vi "senser.vi"(1 "read buffer":string) -> (0 "输出簇":cluster{"T1":i16, "T2":i16, "T3":i16, "T4":i16})   [LabVIEW 2014]
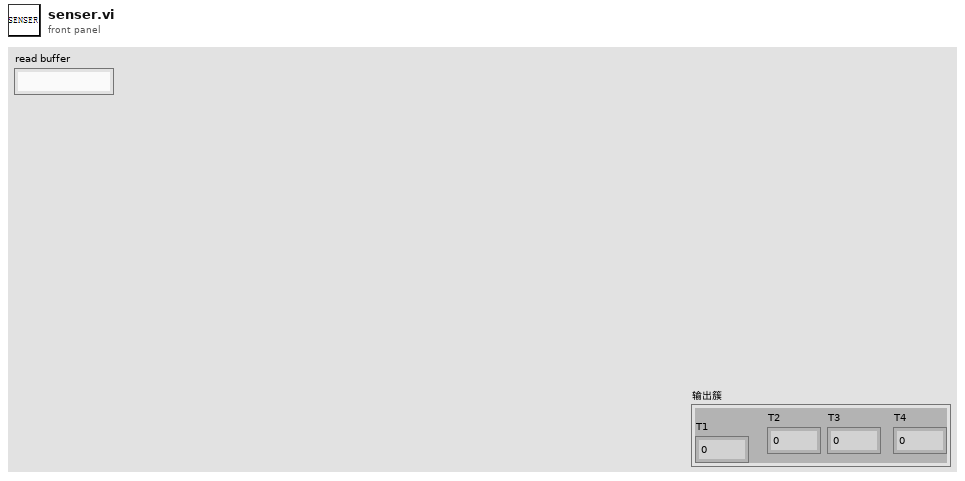
[diagram p1: front panel]
types:
  T1 = cluster{"16位整型":u16, "16位整型":u16, "16位整型":u16, "16位整型":u16}
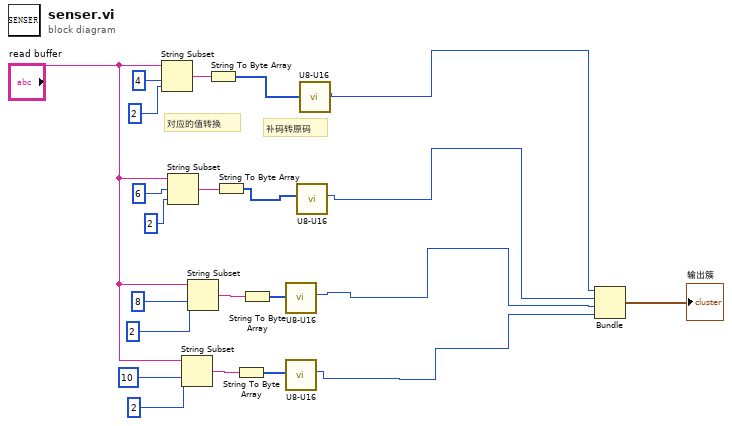
[diagram p0: block diagram]
diagram:
  # "对应的值转换"
  # "补码转原码"
  n1 = String Subset(string="read buffer", offset (0)=4 ("长度（剩余）"), length (rest)=2 ("长度（剩余）")) -> (substring=w12:string)
  n2 = String Subset(string="read buffer", offset (0)=6 ("长度（剩余）"), length (rest)=2 ("长度（剩余）")) -> (substring=w15:string)
  n3 = String Subset(string="read buffer", offset (0)=10 ("长度（剩余）"), length (rest)=2 ("长度（剩余）")) -> (substring=w21:string)
  n4 = String Subset(string="read buffer", offset (0)=8 ("长度（剩余）"), length (rest)=2 ("长度（剩余）")) -> (substring=w18:string)
  n5 = String To Byte Array(string=w12) -> (unsigned byte array=w8:u8[])
  n6 = String To Byte Array(string=w15) -> (unsigned byte array=w6:u8[])
  n7 = String To Byte Array(string=w21) -> (unsigned byte array=w2:u8[])
  n8 = String To Byte Array(string=w18) -> (unsigned byte array=w4:u8[])
  n9 = call "U8-U16.vi"("数组"=w4) -> ("16位整型"=w3:u16)  [unwired: 8 in, 1 out]
  n10 = call "U8-U16.vi"("数组"=w2) -> ("16位整型"=w1:u16)  [unwired: 8 in, 1 out]
  n11 = call "U8-U16.vi"("数组"=w6) -> ("16位整型"=w5:u16)  [unwired: 8 in, 1 out]
  n12 = call "U8-U16.vi"("数组"=w8) -> ("16位整型"=w7:u16)  [unwired: 8 in, 1 out]
  n13 = Bundle("16位整型"=w7, "16位整型"=w5, "16位整型"=w3, "16位整型"=w1) -> (→"输出簇":T1)  [unwired: 1 in]
